vi "Get Model Info - from SysDef.vi"(0 "System Definition Filepath (.nivssdf)":path, 11 "Error (in)":errorcluster) -> (4 "Parameters":string[](array[string]), 6 "Inports":string[](array[string]), 8 "Outports":string[](array[string]), 10 "Models":string[](array[string]), 15 "Error (out)":errorcluster)   [LabVIEW 2016]
uses:
  NationalInstruments.VeriStand.SystemDefinitionAPI
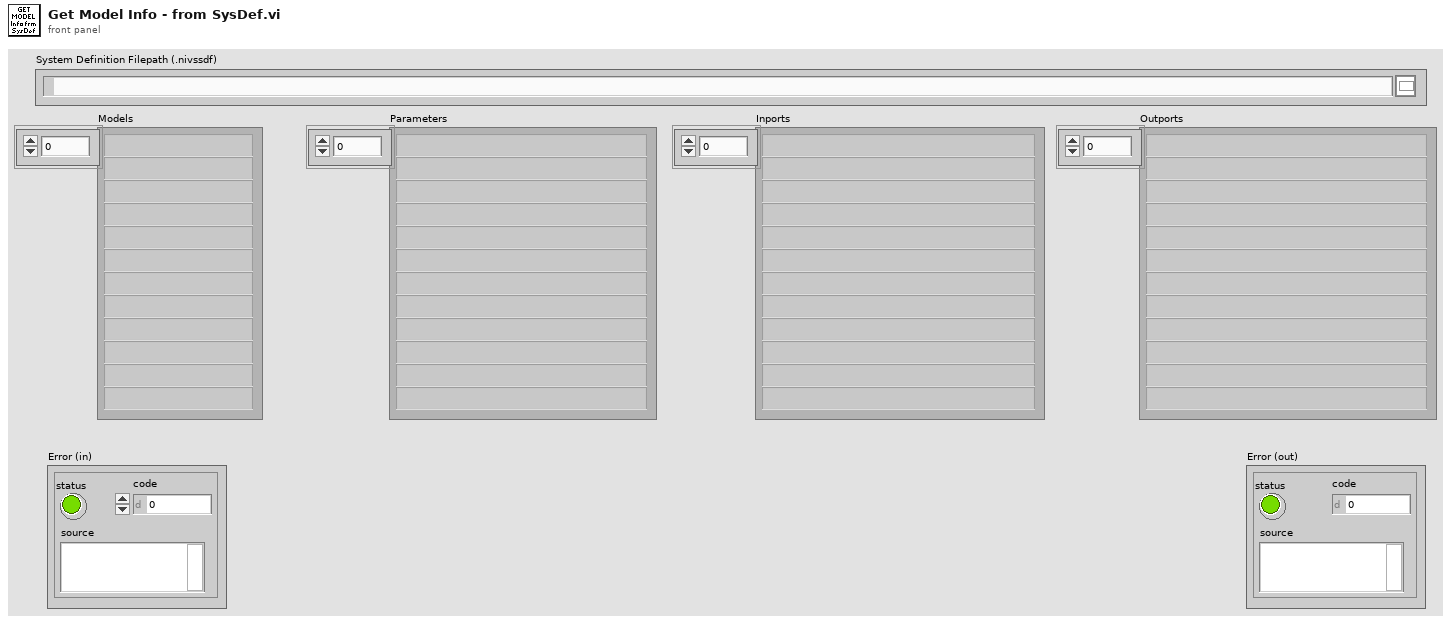
[diagram p1: front panel]
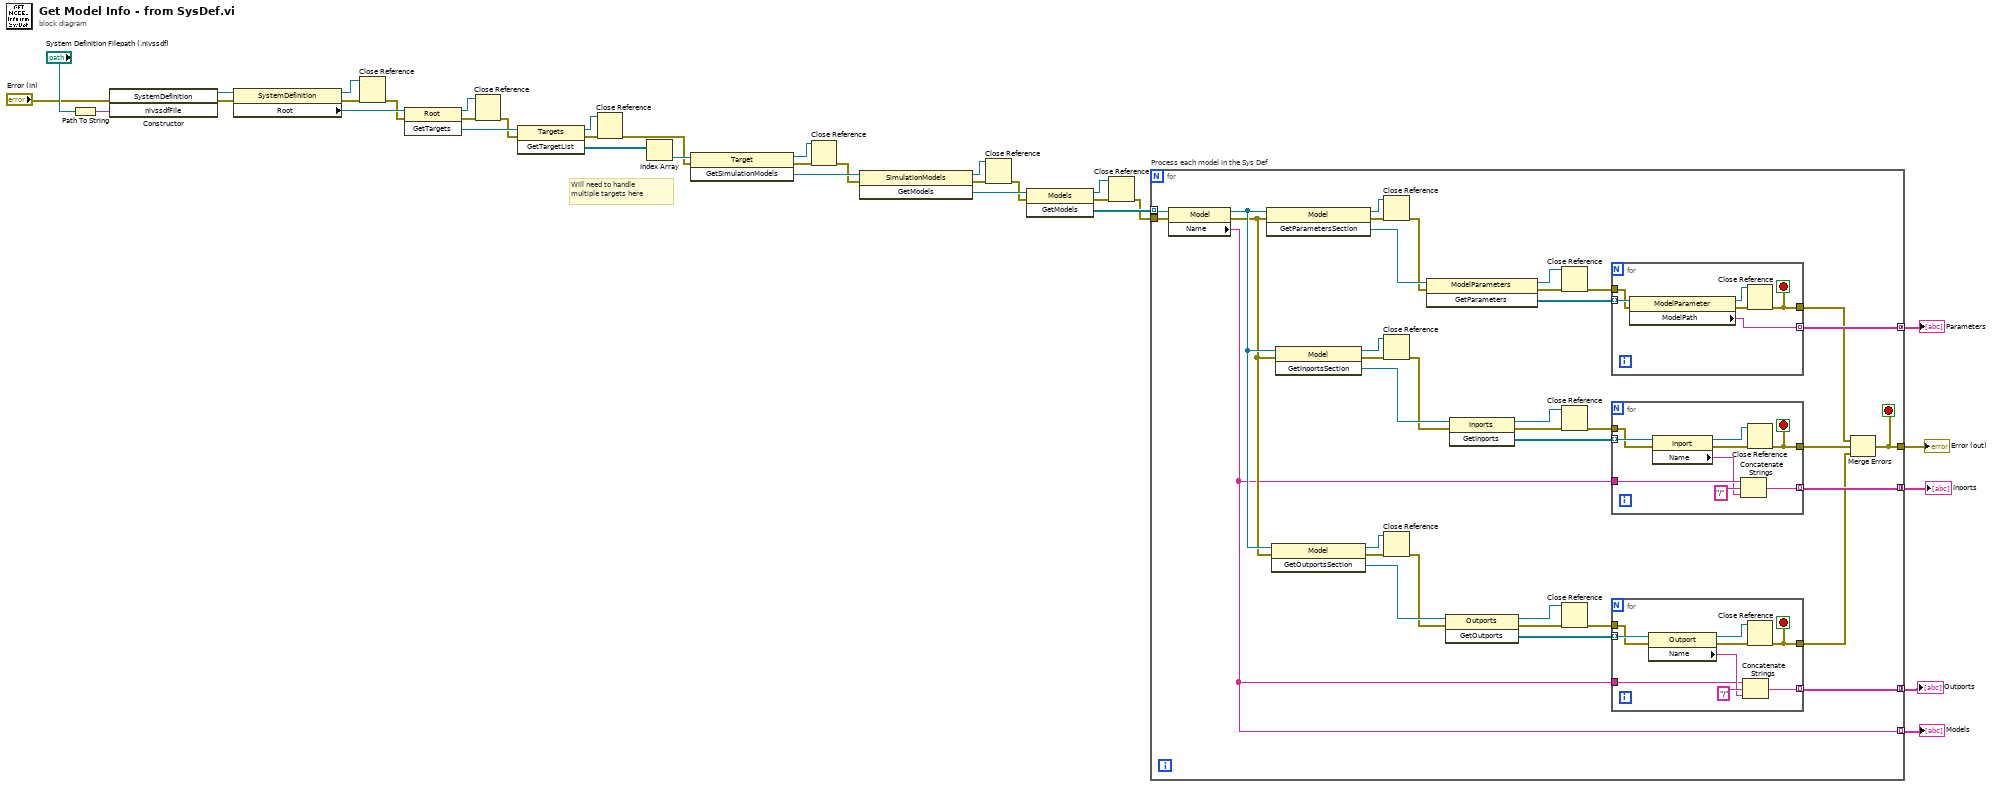
[diagram p0: block diagram]
diagram:
  # "Will need to handle multiple targets here"
  n1 = Path To String(path="System Definition Filepath (.nivssdf)") -> (string=w34:string)
  n2 = constructor class="SystemDefinition"(error in="Error (in)", "nivssdfFile"=w34) -> (reference out=w33:refnum<k24>, error out=w32:errorcluster)  [unwired: 2 in, 2 out]
  n3 = property class="SystemDefinition"(reference=w33, error in=w32) -> (reference out=w23:refnum<k24>, error out=w22:errorcluster, "Root"=w27:refnum<k24>)
  n4 = Close Reference(reference=w23, error in (no error)=w22) -> (error out=w21:errorcluster)
  n5 = invoke class="Root" method="GetTargets"(reference=w27, error in=w21) -> (reference out=w17:refnum<k24>, error out=w20:errorcluster, "GetTargets"=w26:refnum<k24>)  [unwired: 1 in]
  n6 = Close Reference(reference=w17, error in (no error)=w20) -> (error out=w19:errorcluster)
  n7 = invoke class="Targets" method="GetTargetList"(reference=w26, error in=w19) -> (reference out=w15:refnum<k24>, error out=w18:errorcluster, "GetTargetList"=w25:refnum<k24>[])  [unwired: 1 in]
  n8 = Close Reference(reference=w15, error in (no error)=w18) -> (error out=w16:errorcluster)
  n9 = Index Array(array=w25) -> (element=w31:refnum<k24>)  [unwired: 1 in]
  n10 = invoke class="Target" method="GetSimulationModels"(reference=w31, error in=w16) -> (reference out=w12:refnum<k24>, error out=w14:errorcluster, "GetSimulationModels"=w30:refnum<k24>)  [unwired: 1 in]
  n11 = Close Reference(reference=w12, error in (no error)=w14) -> (error out=w13:errorcluster)
  n12 = invoke class="SimulationModels" method="GetModels"(reference=w30, error in=w13) -> (reference out=w9:refnum<k24>, error out=w11:errorcluster, "GetModels"=w29:refnum<k24>)  [unwired: 1 in]
  n13 = Close Reference(reference=w9, error in (no error)=w11) -> (error out=w10:errorcluster)
  n14 = invoke class="Models" method="GetModels"(reference=w29, error in=w10) -> (reference out=w6:refnum<k24>, error out=w8:errorcluster, "GetModels"=w28:refnum<k24>[])  [unwired: 1 in]
  n15 = Close Reference(reference=w6, error in (no error)=w8) -> (error out=w7:errorcluster)
  n16 = for "Process each model in the Sys Def" {
    tunnel: w28 -> [w70] mode=indexing
    tunnel: w7 -> [w71]
    tunnel: [w67] -> w24 mode=concatenating
    tunnel: [w36] -> w5 mode=indexing
    tunnel: [w37] -> w4
    tunnel: [w42] -> w2 mode=concatenating
    tunnel: [w41] -> w1 mode=concatenating
    stop <- w37 stop-if-true
    n17 = property class="Model"(reference=w70, error in=w71) -> (reference out=w44:refnum<k24>, error out=w43:errorcluster, "Name"=w36:string)
    n18 = invoke class="Model" method="GetParametersSection"(reference=w44, error in=w43) -> (reference out=w65:refnum<k24>, error out=w66:errorcluster, "GetParametersSection"=w69:refnum<k24>)  [unwired: 1 in]
    n19 = invoke class="Model" method="GetOutportsSection"(reference=w44, error in=w43) -> (reference out=w49:refnum<k24>, error out=w50:errorcluster, "GetOutportsSection"=w52:refnum<k24>)  [unwired: 1 in]
    n20 = invoke class="Model" method="GetInportsSection"(reference=w44, error in=w43) -> (reference out=w57:refnum<k24>, error out=w58:errorcluster, "GetInportsSection"=w60:refnum<k24>)  [unwired: 1 in]
    n21 = Close Reference(reference=w65, error in (no error)=w66) -> (error out=w64:errorcluster)
    n22 = Close Reference(reference=w57, error in (no error)=w58) -> (error out=w56:errorcluster)
    n23 = Close Reference(reference=w49, error in (no error)=w50) -> (error out=w48:errorcluster)
    n24 = invoke class="ModelParameters" method="GetParameters"(reference=w69, error in=w64) -> (reference out=w61:refnum<k24>, error out=w63:errorcluster, "GetParameters"=w68:refnum<k24>[])  [unwired: 1 in]
    n25 = invoke class="Outports" method="GetOutports"(reference=w52, error in=w48) -> (reference out=w45:refnum<k24>, error out=w47:errorcluster, "GetOutports"=w51:refnum<k24>[])  [unwired: 1 in]
    n26 = invoke class="Inports" method="GetInports"(reference=w60, error in=w56) -> (reference out=w53:refnum<k24>, error out=w55:errorcluster, "GetInports"=w59:refnum<k24>[])  [unwired: 1 in]
    n27 = Close Reference(reference=w61, error in (no error)=w63) -> (error out=w62:errorcluster)
    n28 = Close Reference(reference=w53, error in (no error)=w55) -> (error out=w54:errorcluster)
    n29 = Close Reference(reference=w45, error in (no error)=w47) -> (error out=w46:errorcluster)
    n30 = for {
      tunnel: w68 -> [w95] mode=indexing
      tunnel: [w90] -> w67 mode=indexing
      tunnel: w62 -> [w94]
      tunnel: [w92] -> w40
      stop <- w92 stop-if-true
      n31 = property class="ModelParameter"(reference=w95, error in=w94) -> (reference out=w91:refnum<k24>, error out=w93:errorcluster, "ModelPath"=w90:string)
      n32 = Close Reference(reference=w91, error in (no error)=w93) -> (error out=w92:errorcluster)
    }
    n33 = for {
      tunnel: w59 -> [w89] mode=indexing
      tunnel: [w81] -> w42 mode=indexing
      tunnel: w54 -> [w88]
      tunnel: [w86] -> w39
      tunnel: w36 -> [w83]
      stop <- w86 stop-if-true
      n34 = property class="Inport"(reference=w89, error in=w88) -> (reference out=w85:refnum<k24>, error out=w87:errorcluster, "Name"=w82:string)
      n35 = Concatenate Strings(w83, "/" ("string"), w82) -> (w81:string)
      n36 = Close Reference(reference=w85, error in (no error)=w87) -> (error out=w86:errorcluster)
    }
    n37 = for {
      tunnel: w51 -> [w80] mode=indexing
      tunnel: [w73] -> w41 mode=indexing
      tunnel: w46 -> [w79]
      tunnel: [w77] -> w38
      tunnel: w36 -> [w72]
      stop <- w77 stop-if-true
      n38 = property class="Outport"(reference=w80, error in=w79) -> (reference out=w76:refnum<k24>, error out=w78:errorcluster, "Name"=w74:string)
      n39 = Concatenate Strings(w72, "/" ("string"), w74) -> (w73:string)
      n40 = Close Reference(reference=w76, error in (no error)=w78) -> (error out=w77:errorcluster)
    }
    n41 = Merge Errors(w40, w39, w38) -> (w37:errorcluster)
  }
  "Models" <- w5
  "Error (out)" <- w4
  "Parameters" <- w24
  "Inports" <- w2
  "Outports" <- w1
